vi "FindStateInArray.vi"(9 "TransactionState":string, 10 "AllCaseStates":string[](array[string])) -> (1 "CaseStateOut":string, 2 "index of element":i32, 3 "AllIndexes":i32[](array[numeric]))   [LabVIEW 2020, in "StateReverse.lvclass"]
uses:
  <resource>/Framework/Providers/Open_GDS/UML/StateReverse_class/StateReverse.lvclass
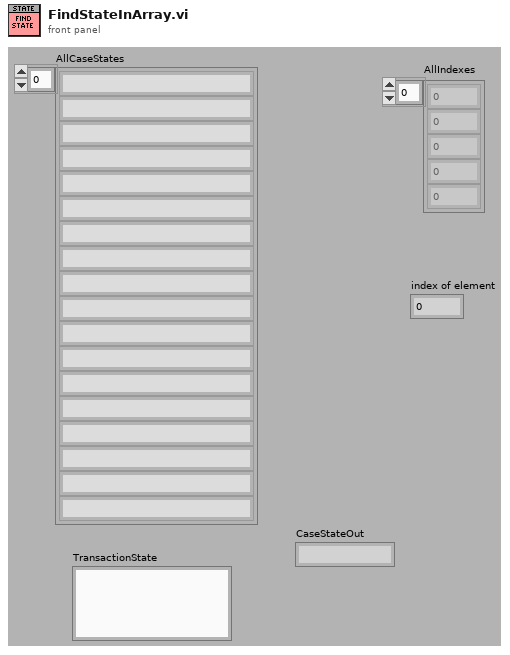
[diagram p1: front panel]
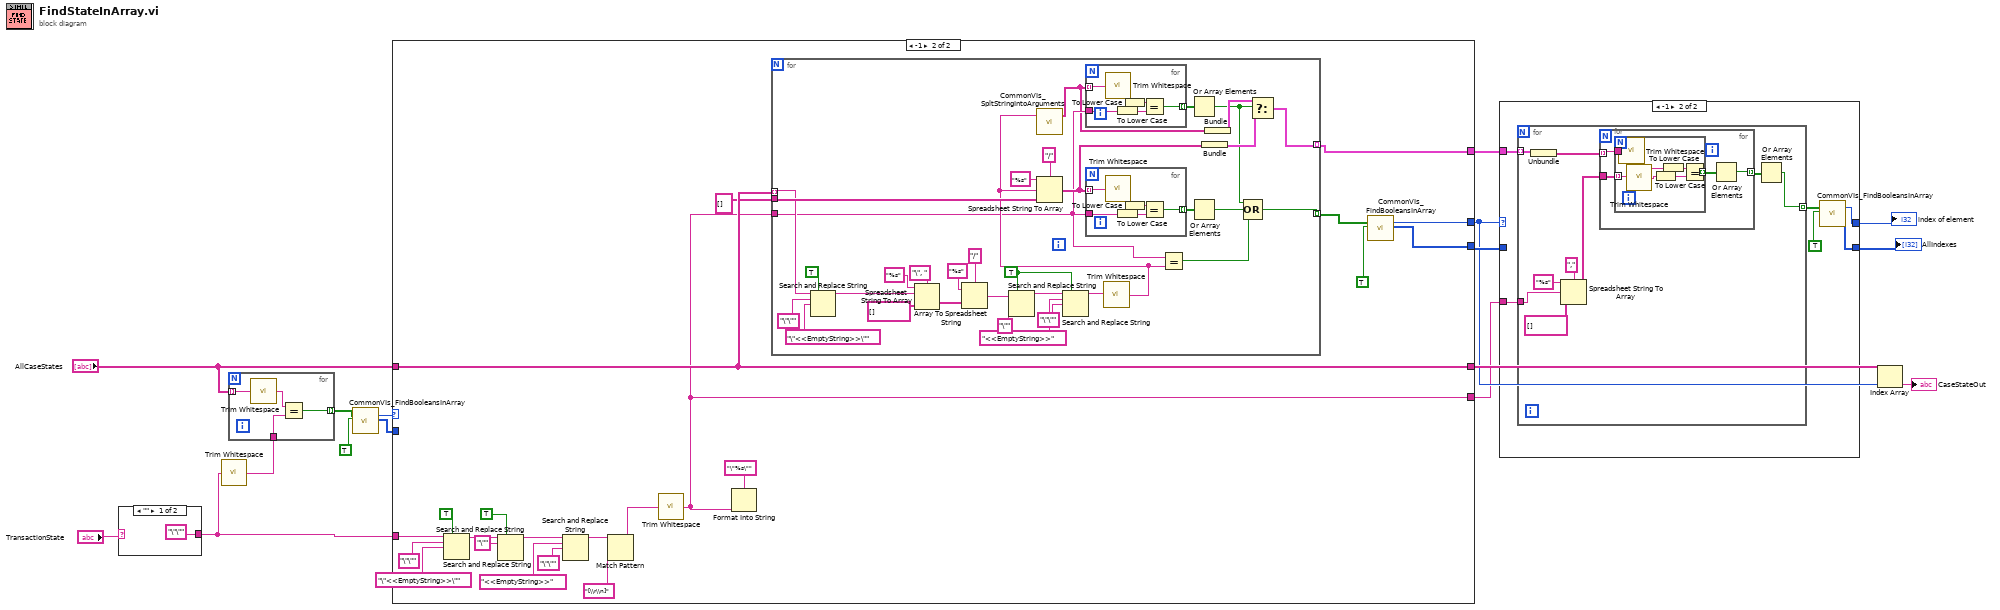
[diagram p0: block diagram]
diagram:
  n1 = case shown="\"\"" "TransactionState" {
    selector: "TransactionState" -> [_ w18]
    tunnel: ["\"\"" ("delimiter (Tab)") w18] -> w15
    frame "" {
    }
    frame Default {
    }
  }
  n2 = call <vilib>:"Trim Whitespace.vi"("string"=w15) -> ("trimmed string"=w10:string)  [unwired: 1 in]
  n3 = for {
    tunnel: "AllCaseStates" -> [w22] mode=indexing
    tunnel: w10 -> [w20]
    tunnel: [w19] -> w9 mode=indexing
    n4 = call <vilib>:"Trim Whitespace.vi"("string"=w22) -> ("trimmed string"=w21:string)  [unwired: 1 in]
    n5 = Equal?(x=w21, y=w20) -> (x = y?=w19:bool)
  }
  n6 = call <resource>:"CommonVIs_FindBooleansInArray.vi"("1D array"=w9, "element"=TRUE) -> ("index of element"=w8:i32, "ArrayOfIndexOfElement"=w7:i32[])  [unwired: 16 out]
  n7 = case shown="-1" w8 {
    selector: w8 -> [w24 _]
    tunnel: [w24 w36] -> w5
    tunnel: [w23 w35] -> w6
    tunnel: w15 -> [_ w31]
    tunnel: "AllCaseStates" -> [w25 w30]
    tunnel: [w25 w30] -> w13
    tunnel: w7 -> [w23 _]
    tunnel: [_ w27] -> w2
    tunnel: [_ w26] -> w1
    frame 0, Default {
    }
    frame -1 {
      n8 = Search and Replace String(replace all?=TRUE ("replace all? (F)"), input string=w31, search string="\"\"" ("delimiter (Tab)"), replace string="\"<<EmptyString>>\"" ("delimiter (Tab)")) -> (result string=w41:string)  [unwired: 4 in, 3 out]
      n9 = Search and Replace String(replace all?=TRUE ("replace all? (F)"), input string=w41, search string="\"") -> (result string=w39:string)  [unwired: 5 in, 3 out]
      n10 = Search and Replace String(input string=w39, search string="<<EmptyString>>" ("delimiter (Tab)"), replace string="\"\"" ("delimiter (Tab)")) -> (result string=w34:string)  [unwired: 5 in, 3 out]
      n11 = Match Pattern(string=w34, regular expression="[\\r\\n]") -> (before substring=w32:string)  [unwired: 1 in, 3 out]
      n12 = call <vilib>:"Trim Whitespace.vi"("string"=w32) -> ("trimmed string"=w26:string)  [unwired: 1 in]
      n13 = Format Into String(format string="\"%s\"", w26) -> ()  [unwired: 2 in, 2 out]
      n14 = for {
        tunnel: w30 -> [w59] mode=indexing
        tunnel: [w57] -> w28 mode=indexing
        tunnel: string[] [] -> [w80]
        tunnel: w26 -> [w53]
        tunnel: [w49] -> w27 mode=indexing
        w64 = TRUE ("replace all? (F)")
        n15 = Search and Replace String(replace all?=TRUE ("replace all? (F)"), input string=w59, search string="\"\"" ("delimiter (Tab)"), replace string="\"<<EmptyString>>\"" ("delimiter (Tab)")) -> (result string=w67:string)  [unwired: 1 in, 6 out]
        n16 = Spreadsheet String To Array(delimiter (Tab)="\", ", format string="%s", spreadsheet string=w67, array type (2D Dbl)=string[] []) -> (array=w73:string[])
        n17 = Array To Spreadsheet String(delimiter (Tab)="/", array=w73, 3:"%s" ("format string")) -> (spreadsheet string=w70:string)
        n18 = Search and Replace String(replace all?=w64, input string=w70, search string="\"" ("delimiter (Tab)")) -> (result string=w65:string)  [unwired: 1 in, 7 out]
        n19 = Search and Replace String(replace all?=w64, input string=w65, search string="<<EmptyString>>" ("delimiter (Tab)"), replace string="\"\"" ("delimiter (Tab)")) -> (result string=w60:string)  [unwired: 1 in, 6 out]
        n20 = call <vilib>:"Trim Whitespace.vi"("string"=w60) -> ("trimmed string"=w55:string)  [unwired: 1 in]
        n21 = call <resource>:"CommonVIs_SpltStringIntoArguments.vi"("String"=w55) -> ("splittedString"=w52:string[])  [unwired: 17 in, 1 out]
        n22 = Spreadsheet String To Array(delimiter (Tab)="/", format string="%s", spreadsheet string=w55, array type (2D Dbl)=w80) -> (array=w56:string[])
        n23 = for {
          tunnel: w52 -> [w84] mode=indexing
          tunnel: w53 -> [w87]
          tunnel: [w86] -> w54 mode=indexing
          n24 = call <vilib>:"Trim Whitespace.vi"("string"=w84) -> ("trimmed string"=w85:string)  [unwired: 1 in]
          n25 = To Lower Case(string=w87) -> (all lower case string=w82:string)
          n26 = To Lower Case(string=w85) -> (all lower case string=w83:string)
          n27 = Equal?(x=w83, y=w82) -> (x = y?=w86:bool)
        }
        n28 = for {
          tunnel: w56 -> [w90] mode=indexing
          tunnel: w53 -> [w93]
          tunnel: [w92] -> w78 mode=indexing
          n29 = call <vilib>:"Trim Whitespace.vi"("string"=w90) -> ("trimmed string"=w91:string)  [unwired: 1 in]
          n30 = To Lower Case(string=w93) -> (all lower case string=w88:string)
          n31 = To Lower Case(string=w91) -> (all lower case string=w89:string)
          n32 = Equal?(x=w89, y=w88) -> (x = y?=w92:bool)
        }
        n33 = Equal?(x=w53, y=w55) -> (x = y?=w58:bool)
        n34 = Or Array Elements(Boolean array=w54) -> (logical OR=w48:bool)
        n35 = Or Array Elements(Boolean array=w78) -> (logical OR=w77:bool)
        n36 = Bundle(w56) -> (w50:cluster{string[]})  [unwired: 1 in]
        n37 = Bundle("splittedString"=w52) -> (w51:cluster{"splittedString":string[]})  [unwired: 1 in]
        n38 = Compound Arithmetic op=OR(w48, w77, w58) -> (w57:bool)
        n39 = Select(t=w51, s=w48, f=w50) -> (s? t:f=w49:cluster{"splittedString":string[]})
      }
      n40 = call <resource>:"CommonVIs_FindBooleansInArray.vi"("1D array"=w28, "element"=TRUE) -> ("index of element"=w36:i32, "ArrayOfIndexOfElement"=w35:i32[])  [unwired: 16 out]
    }
  }
  n41 = case shown="-1" w5 {
    selector: w5 -> [w95 _]
    tunnel: [w95 w97] -> w3
    tunnel: [w94 w96] -> w4
    tunnel: w6 -> [w94 _]
    tunnel: w2 -> [_ w100]
    tunnel: w1 -> [_ w101]
    frame 0, Default {
    }
    frame -1 {
      n42 = for {
        tunnel: w101 -> [w104]
        tunnel: w100 -> [w108] mode=indexing
        tunnel: [w102] -> w99 mode=indexing
        n43 = Unbundle(w108) -> ("splittedString"=w106:string[])
        n44 = Spreadsheet String To Array(delimiter (Tab)=",", format string="%s", spreadsheet string=w104, array type (2D Dbl)=string[] []) -> (array=w107:string[])
        n45 = for {
          tunnel: w106 -> [w113] mode=indexing
          tunnel: w107 -> [w114]
          tunnel: [w111] -> w105 mode=indexing
          n46 = for {
            tunnel: w114 -> [w116] mode=indexing
            tunnel: [w121] -> w112 mode=indexing
            tunnel: w113 -> [w119]
            n47 = call <vilib>:"Trim Whitespace.vi"("string"=w119) -> ("trimmed string"=w120:string)  [unwired: 1 in]
            n48 = call <vilib>:"Trim Whitespace.vi"("string"=w116) -> ("trimmed string"=w115:string)  [unwired: 1 in]
            n49 = To Lower Case(string=w115) -> (all lower case string=w117:string)
            n50 = To Lower Case(string=w120) -> (all lower case string=w118:string)
            n51 = Equal?(x=w118, y=w117) -> (x = y?=w121:bool)
          }
          n52 = Or Array Elements(Boolean array=w112) -> (logical OR=w111:bool)
        }
        n53 = Or Array Elements(Boolean array=w105) -> (logical OR=w102:bool)
      }
      n54 = call <resource>:"CommonVIs_FindBooleansInArray.vi"("1D array"=w99, "element"=TRUE) -> ("index of element"=w97:i32, "ArrayOfIndexOfElement"=w96:i32[])  [unwired: 16 out]
    }
  }
  "index of element" <- w3
  "AllIndexes" <- w4
  n55 = Index Array(array=w13, index=w5) -> (element=→"CaseStateOut":string)
